vi "To Pythonic - Integer Array.vi"(4 "Integer Array":i64[](array[numeric])) -> (1 "Pythonic Value":string)   [LabVIEW 2020, in "OPI.lvclass"]
doc: "Convert LabVIEW data into valid pythonic representation."
uses:
  OPI.lvclass
  <vilib>/AdvancedString/Join Strings.vi
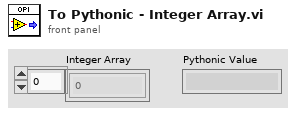
[diagram p1: front panel]
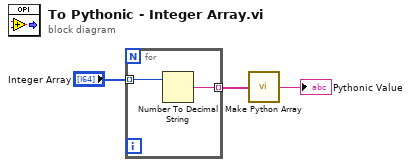
[diagram p0: block diagram]
diagram:
  n1 = for {
    tunnel: "Integer Array" -> [w5] mode=indexing
    tunnel: [w4] -> w2 mode=indexing
    n2 = Number To Decimal String(number=w5) -> (decimal integer string=w4:string)  [unwired: 1 in]
  }
  n3 = call "Make Python Array.vi"("Pythonic Values"=w2) -> ("Pythonic Array"=→"Pythonic Value":string)
